vi "Queue Periodic Updates.vi"(10 "Last Periodic Update in":u32, 11 "Remaining States":string) -> (2 "Last Periodic Update out":u32, 3 "States Out":string)   [LabVIEW 2023]
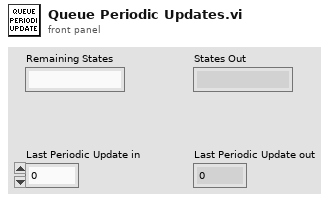
[diagram p1: front panel]
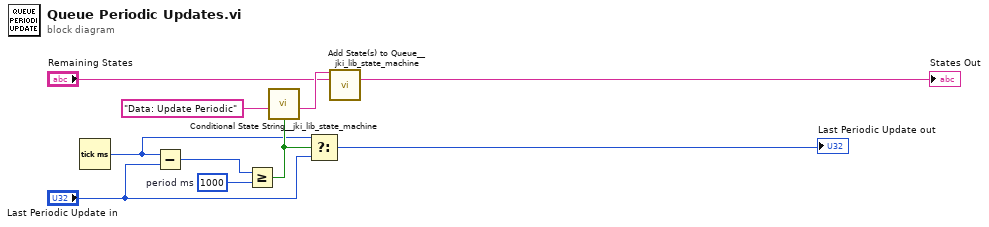
[diagram p0: block diagram]
diagram:
  w9 = u32 1000  # period ms
  n1 = Tick Count (ms)() -> (millisecond timer value=w6:u32)
  n2 = Subtract(x=w6, y="Last Periodic Update in") -> (x-y=w7:u32)
  n3 = Greater Or Equal?(x=w7, y=w9) -> (x >= y?=w8:bool)
  n4 = call <vilib>:"Conditional State String__jki_lib_state_machine.vi"("Do State(s)?"=w8, "State"="Data: Update Periodic") -> ("State Out"=w4:string)  [unwired: 7 in]
  n5 = Select(t=w6, s=w8, f="Last Periodic Update in") -> (s? t:f=→"Last Periodic Update out":u32)
  n6 = call <vilib>:"Add State(s) to Queue__jki_lib_state_machine.vi"("State(s) in Front (\"\")"=w4, "State(s) in (\"\")"="Remaining States") -> ("States Out"=→"States Out":string)  [unwired: 13 in]
